vi "SET_SHOOTER_SPEED.vi"(10 "argv":string[](array[string]), 11 "args":u8) -> ()   [LabVIEW 2015]
uses:
  Team Code/Robot Global Data.vi
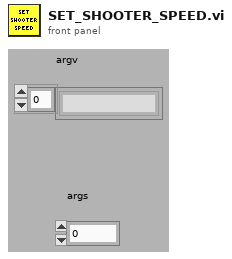
[diagram p1: front panel]
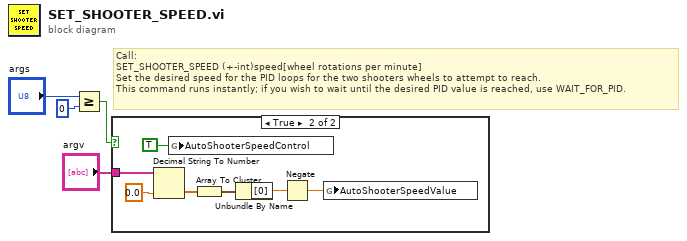
[diagram p0: block diagram]
diagram:
  # "Call:\nSET_SHOOTER_SPEED (+-int)speed[wheel rotations per minute]\nSet the desired speed for the PID loops for the two shooters wheels to attempt to reach.\nThis command runs instantly; if you wish to wait until the desired PID value is reached, use WAIT_FOR_PID."
  n1 = Greater Or Equal?(x="args", y=u8 0) -> (x >= y?=w4:bool)
  n2 = case shown="True" w4 {
    tunnel: "argv" -> [_ w11]
    frame False {
    }
    frame True {
      n3 = Decimal String To Number(string=w11, default (0L)=0.0 ("default (0 I32)")) -> (number=w9:dbl[])  [unwired: 2 out]
      n4 = global write "Robot Global Data.vi" "AutoShooterSpeedControl"(TRUE ("AutoArmControl")) -> ()
      n5 = Array To Cluster(array=w9) -> (cluster=w8:cluster{"[0]":dbl, "[1]":dbl})
      n6 = Unbundle By Name(w8) -> ("[0]"=w6:dbl)
      n7 = Negate(x=w6) -> (-x=w5:dbl)
      n8 = global write "Robot Global Data.vi" "AutoShooterSpeedValue"(w5) -> ()
    }
  }
